vi "VirtualBigAccDAQ.vi"() -> ()   [LabVIEW 2013]
uses:
  <vilib>/Utility/miscctls.llb/LVPointTypeDef.ctl
  Database2.0/Public API/Dust_Event.ctl
  Database2.0/Public API/Signal.ctl
  Database2.0/Private/Controls/Role ID.ctl
  Database2.0/Private/Controls/Hardware ID.ctl
  Database2.0/Private/Controls/Estimate_source.ctl
  <userlib>/_OpenG.lib/numeric/numeric.llb/Random Number Within Range - I32__ogtk.vi
  <vilib>/measure/mamon.llb/Trigger Detection for 1 Channel.vi
  Database2.0/Private/UI Elements/PSU updated.vi
  <userlib>/_OpenG.lib/comparison/comparison.llb/DBL Changed__ogtk.vi
  <vilib>/measure/NI_MAPro.lvlib
panel:
  out "Random":bool
  in  "User Select":bool
  in  "User Selected Dust ID":i32=2633939
  out "Original Dust ID":i32
  in  "Read new file":bool
  out "Detectors 1 and 2":waveform(dbl)[](graph)
  in  "Write to Database?":bool
  out "PSU":waveform(dbl)(graph)
  out "Detector 3":waveform(dbl)(graph)
  out "Avg. Rate":dbl format="%#.3g"
  in  "Reset Count":bool
  in  "min sample rate":dbl=1000000.0 format="%.2p"
  in  "Clear Errors?":bool
  out "No. of Events":i32
  out "error out":errorcluster
  in  "stop":bool
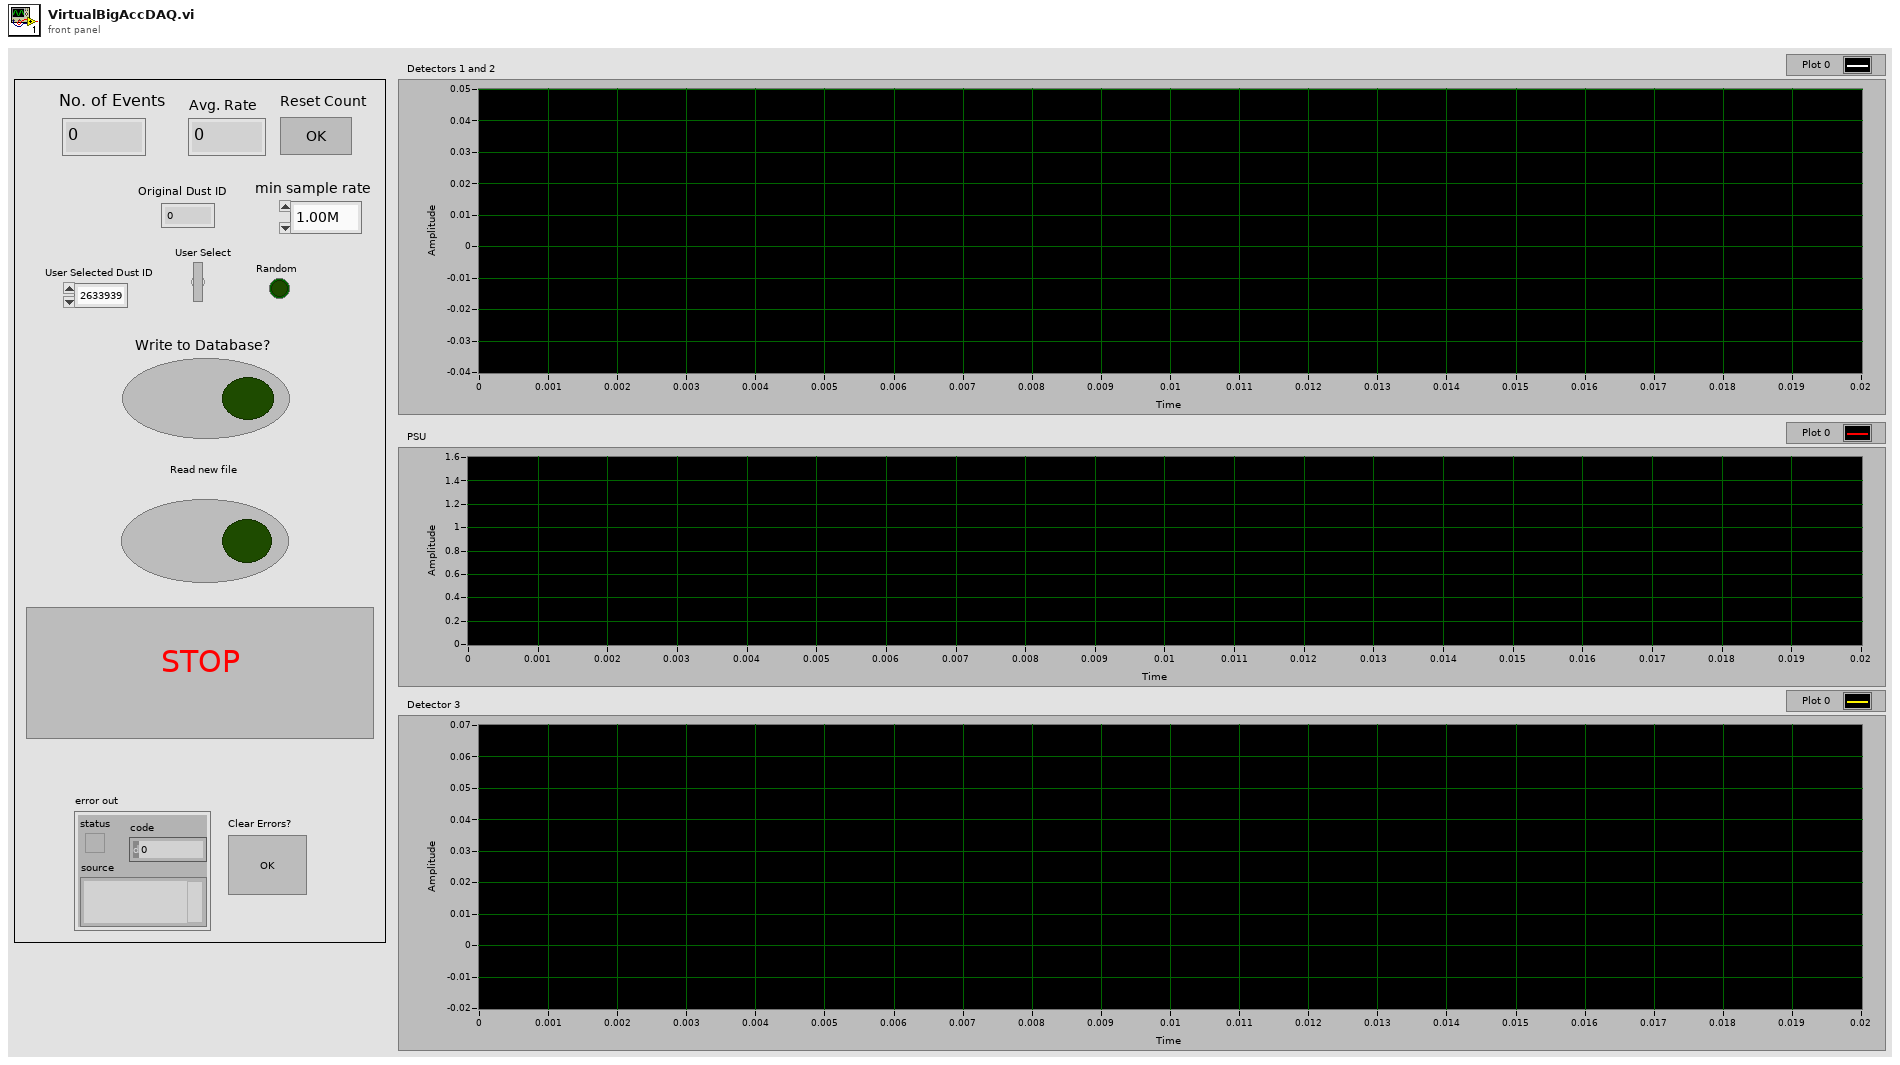
[diagram p1: front panel]
types:
  T1 = typedef "LVPointTypeDef.ctl" = cluster{"Horizontal":i16, "Vertical":i16}
  T2 = cluster{"relativeInitialX":dbl, "xIncrement":dbl, "wfm":dbl[]}
  T3 = typedef "Dust_Event.ctl" = cluster{"Time Stamp":timestamp, "Velocity":sgl, "Mass":sgl, "Charge":sgl, "Radius":sgl, "Array":T4[], "Dust Event ID":i64, "Passed_3rd_Detector":bool, "Estimate Source":T7, "Estimate Quality":sgl}
  T4 = typedef "Signal.ctl" = cluster{"Signal ID":i64, "Time Stamp":timestamp, "Dust Event ID":i64, "Role ID":T5, "Data":sgl[], "Signal Length":i32, "dt":sgl, "Offset":dbl, "Hardware ID":T6}
  T5 = typedef "Role ID.ctl" = enum16{"First_Detector", "Second_Detector", "Third_Detector", "LeCroy_CH1", "LeCroy_CH2", "LeCroy_CH3", "LeCroy_CH4", "PSU"}
  T6 = typedef "Hardware ID.ctl" = enum16{"Unknown", "CSA 1", "CSA 2", "CSA 3", "CSA 4", "CSA 5", "CSA 6"}
  T7 = typedef "Estimate_source.ctl" = i8
  T8 = typedef "Waveforms.ctl" = cluster{"id_dust_event":u64, "Time Stamp":timestamp, "Velocity":dbl, "Mass":dbl, "Charge":dbl, "Radius":dbl, "Waveform Graph":sgl[][], "Quality":i32}
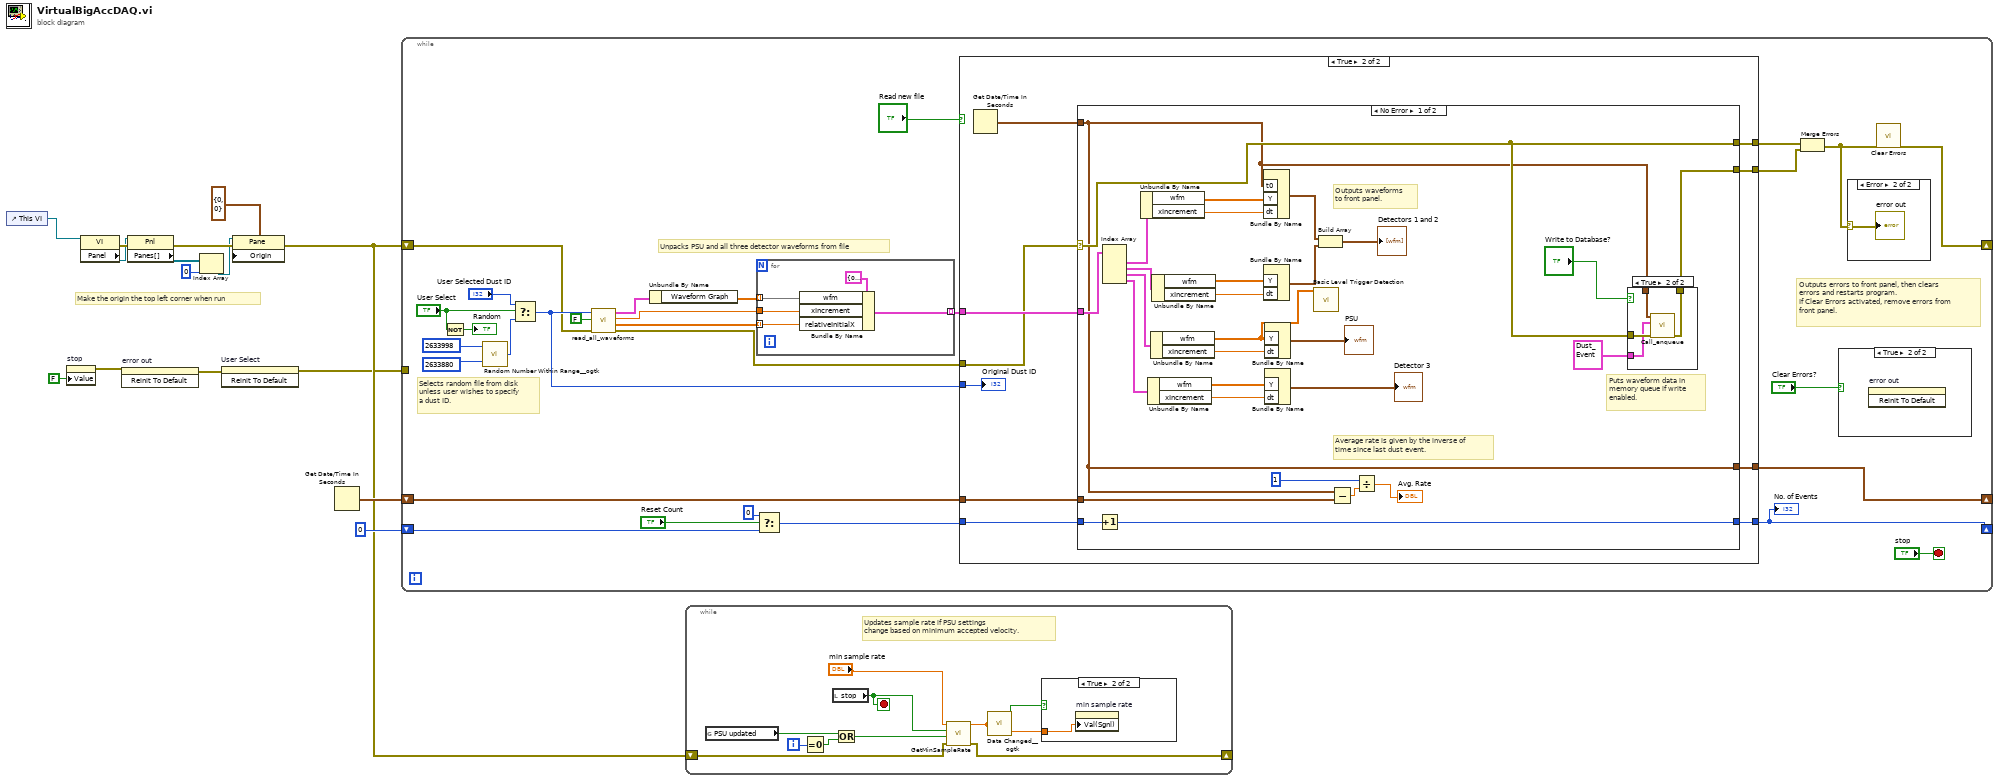
[diagram p0: block diagram]
diagram:
  # "Make the origin the top left corner when run"
  n1 = control-ref of="This VI"() -> (w8:refnum<vi>)
  n2 = property on="stop" class="Bool (strict)"("Value"=FALSE ("stop")) -> (error out=w5:errorcluster)  [unwired: 2 in, 1 out]
  n3 = property class="VI"(reference=w8) -> (error out=w15:errorcluster, "Panel"=w9:refnum<vi>)  [unwired: 1 in, 1 out]
  n4 = invoke on="error out" class="Clust (strict)" method="Reinit To Default"(error in=w5) -> (error out=w2:errorcluster)  [unwired: 2 in, 2 out]
  n5 = property class="Pnl"(reference=w9, error in=w15) -> (error out=w14:errorcluster, "Panes[]"=w13:refnum<vi>[])  [unwired: 1 out]
  n6 = Index Array(array=w13, index=0) -> (element=w11:refnum<vi>)
  n7 = invoke on="User Select" class="Bool (strict)" method="Reinit To Default"(error in=w2) -> (error out=w1:errorcluster)  [unwired: 2 in, 2 out]
  n8 = property class="Pane"(reference=w11, error in=w14, "Origin"=T1 {"Horizontal"=0, "Vertical"=0}) -> (error out=w3:errorcluster)  [unwired: 1 out]
  n9 = Get Date/Time In Seconds() -> (seconds since 1Jan1904=w4:timestamp)
  n10 = while {
    shift-right: [w42] -> _
    shift-left: w3 -> [w19]
    shift-right: [w20] -> _
    shift-left: 0 -> [w36]
    shift-right: [w37] -> _
    shift-left: w4 -> [w39]
    tunnel: w1 -> [_]
    stop <- "stop" stop-if-true
    # "Unpacks PSU and all three detector waveforms from file"
    # "Selects random file from disk\nunless user wishes to specify\na dust ID."
    # "Outputs errors to front panel, then clears \nerrors and restarts program. \nIf Clear Errors activated, remove errors from \nfront panel."
    n11 = Not(x="User Select") -> (.not. x?=→"Random":bool)
    n12 = call-poly <userlib>:"Random Number Within Range__ogtk.vi"("High"=2633998, "Low"=2633880) -> ("Random Number"=w24:i32)  [unwired: 3 in]
    n13 = Select(t="User Selected Dust ID", s="User Select", f=w24) -> (s? t:f=w25:i32)
    n14 = call "read_all_waveforms.vi"("error in (no error)"=w19, "Small?"=FALSE, "Dust Event ID"=w25) -> ("error out"=w18:errorcluster, "Offset Array"=w32:dbl[], "dt"=w33:dbl, "Waveform"=w30:T8)  [unwired: 5 in]
    n15 = Unbundle By Name(w30) -> ("Waveform Graph"=w31:sgl[][])
    n16 = for {
      tunnel: w31 -> [w48] mode=indexing
      tunnel: w32 -> [w46] mode=indexing
      tunnel: w33 -> [w47]
      tunnel: [w45] -> w28 mode=indexing
      n17 = Bundle By Name(cluster=T2 {"relativeInitialX"=0.0, "xIncrement"=0.0, "wfm"=[]}, "wfm"=w48, "xIncrement"=w47, "relativeInitialX"=w46) -> (w45:T2)
    }
    n18 = Select(t=0, s="Reset Count", f=w36) -> (s? t:f=w38:i32)
    n19 = case shown="True" "Read new file" {
      tunnel: [w50 w58] -> w35
      tunnel: [w50 w59] -> w34
      tunnel: w39 -> [w51 w62]
      tunnel: w38 -> [w52 w61]
      tunnel: [w52 w60] -> w20
      tunnel: [w51 w57] -> w37
      tunnel: w28 -> [_ w56]
      tunnel: w25 -> [_ w55]
      tunnel: w18 -> [w50 w53]
      frame False {
      }
      frame True {
        n20 = Get Date/Time In Seconds() -> (seconds since 1Jan1904=w54:timestamp)
        n21 = case shown="No Error" w53 {
          selector: w53 -> [w83 w99]
          tunnel: [w85 w99] -> w58
          tunnel: w61 -> [w84 w98]
          tunnel: [w78 w98] -> w60
          tunnel: [w83 w99] -> w59
          tunnel: w62 -> [w69 w97]
          tunnel: [w64 w97] -> w57
          tunnel: w56 -> [w65 _]
          tunnel: w54 -> [w64 _]
          frame No Error {
            # "Puts waveform data in\nmemory queue if write \nenabled."
            # "Outputs waveforms\nto front panel."
            # "Average rate is given by the inverse of \ntime since last dust event."
            n22 = Increment(x=w84) -> (x+1=w78:i32)
            n23 = Index Array(array=w65) -> (element #1=w91:T2, element #2=w90:T2, element #3=w82:T2, element #4=w81:T2)  [unwired: 4 in]
            n24 = Unbundle By Name(w91) -> ("wfm"=w76:dbl[], "xIncrement"=w75:dbl)
            n25 = Unbundle By Name(w81) -> ("wfm"=w72:dbl[], "xIncrement"=w71:dbl)
            n26 = Unbundle By Name(w82) -> ("wfm"=w63:dbl[], "xIncrement"=w70:dbl)
            n27 = Unbundle By Name(w90) -> ("wfm"=w74:dbl[], "xIncrement"=w73:dbl)
            n28 = Bundle By Name("t0"=w64, "Y"=w76, "dt"=w75) -> (w89:waveform(dbl))  [unwired: 1 in]
            n29 = Bundle By Name("Y"=w74, "dt"=w73) -> (w88:waveform(dbl))  [unwired: 1 in]
            n30 = Bundle By Name("Y"=w63, "dt"=w70) -> (→"PSU":waveform(dbl))  [unwired: 1 in]
            n31 = Bundle By Name("Y"=w72, "dt"=w71) -> (→"Detector 3":waveform(dbl))  [unwired: 1 in]
            n32 = call-poly <vilib>:"Basic Level Trigger Detection.vi"("signal in"=w63) -> ()  [unwired: 12 in, 3 out]
            n33 = Build Array(w89, w88) -> (→"Detectors 1 and 2":waveform(dbl)[])
            n34 = Subtract(x=w64, y=w69) -> (x-y=w67:dbl)
            n35 = Divide(x=1 ("y"), y=w67) -> (x/y=→"Avg. Rate":dbl)
            n36 = case shown="True" "Write to Database?" {
              tunnel: w83 -> [w92 w96]
              tunnel: [w92 w95] -> w85
              tunnel: T3 {"Time Stamp"=timestamp(0 s since 1904-01-01), "Velocity"=0.0, "Mass"=0.0, "Charge"=0.0, "Radius"=0.0, "Array"=[], "Dust Event ID"=0, "Passed_3rd_Detector"=FALSE, "Estimate Source"=0, "Estimate Quality"=0.0} ("Input Data") -> [_ w94]
              tunnel: w64 -> [_ w93]
              frame False {
              }
              frame True {
                n37 = call "Call_enqueue.vi"("error in"=w96, "Input Data"=w94, "Timestamp"=w93) -> ("error out"=w95:errorcluster)  [unwired: 8 in]
              }
            }
          }
          frame Error {
          }
        }
        "Original Dust ID" <- w55
      }
    }
    "No. of Events" <- w20
    n38 = Merge Errors(w34, w35) -> (w44:errorcluster)
    n39 = case shown="True" "Clear Errors?" {
      frame False {
      }
      frame True {
        n40 = invoke on="error out" class="Clust (strict)" method="Reinit To Default"() -> ()  [unwired: 3 in, 3 out]
      }
    }
    n41 = case shown="Error" w44 {
      selector: w44 -> [_ w100]
      frame No Error {
      }
      frame Error {
        "error out" <- w100
      }
    }
    n42 = call <vilib>:"Clear Errors.vi"("error in (no error)"=w44) -> ("error out"=w42:errorcluster)  [unwired: 6 in]
  }
  n43 = while {
    shift-right: [w104] -> _
    shift-left: w3 -> [w107]
    i -> [w110]
    stop <- w105 stop-if-true
    # "Updates sample rate if PSU settings \nchange based on minimum accepted velocity."
    n44 = global read "PSU updated.vi" "PSU updated"() -> (w109:bool)
    n45 = Equal To 0?(x=w110) -> (x = 0?=w108:bool)
    n46 = local read "stop"() -> (w105:bool)
    n47 = Or(x=w109, y=w108) -> (x .or. y?=w106:bool)
    n48 = call "GetMinSampleRate.vi"("error in (no error)"=w107, "PSU Update"=w106, "stop"=w105, "min sample rate"="min sample rate") -> ("error out"=w104:errorcluster, "min sample rate"=w102:dbl)  [unwired: 6 in]
    n49 = call-poly <userlib>:"Data Changed__ogtk.vi"("DBL"=w102) -> ("Changed"=w103:bool)
    n50 = case shown="True" w103 {
      tunnel: w102 -> [_ w111]
      frame False {
      }
      frame True {
        n51 = property on="min sample rate" class="DigNum (strict)"("Val(Sgnl)"=w111) -> ()  [unwired: 2 in, 2 out]
      }
    }
  }
